vi "Stop.vi"(8 "error in (no error)":errorcluster, 10 "Message in":refnum<class "StopMessage.lvclass">, 11 "Autofocus in":refnum<class "Autofocus.lvclass">) -> (0 "error out":errorcluster, 3 "Autofocus out":refnum<class "Autofocus.lvclass">)   [LabVIEW 2012, in "Autofocus.lvclass"]
doc: "This member function is called when the statemachine in the run.vi receives an 'stop' command. It relays the message to all observers of the component.\n\nOverride this member function in your derived class if you need additional stop functionality (but don't forget to call the parent method)."
uses:
  Autofocus.lvclass
  <vilib>/Distrio/Murmex/StopMessage/StopMessage.lvclass
  <vilib>/Distrio/Murmex/Murmex/Murmex.lvclass
  Autofocus.lvclass/Autofocus.ctl
panel:
  out "optimisation duration":dbl
  # "This method is called when the STOP\ntrigger is sent. \n\nOverride this method when your component needs to\nrespond to this trigger. \n\nCall parent for proper implementation"
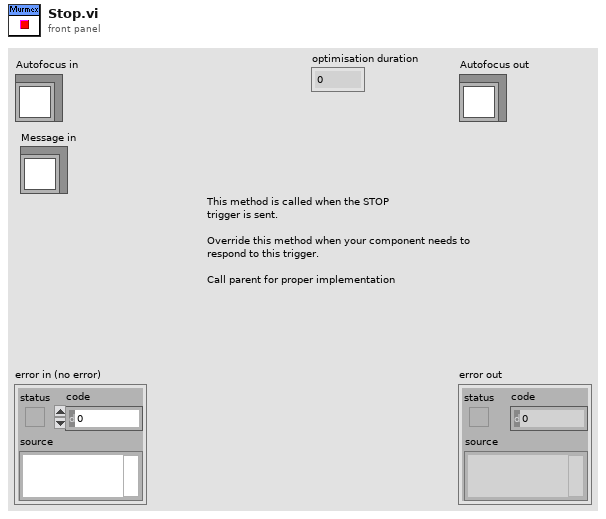
[diagram p1: front panel]
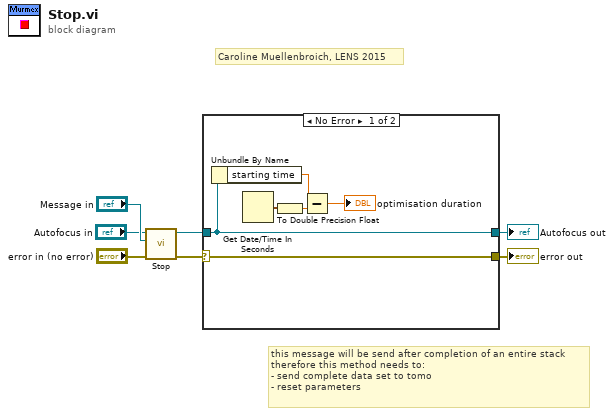
[diagram p0: block diagram]
diagram:
  # "Caroline Muellenbroich, LENS 2015"
  # "this message will be send after completion of an entire stack\ntherefore this method needs to:\n- send complete data set to tomo\n- reset parameters"
  n1 = call-parent "Stop.vi"("error in (no error)"="error in (no error)", "Message in"="Message in", "Murmex in"="Autofocus in") -> ("error out"=w4:errorcluster, "Murmex out"=w3:refnum<class "Autofocus.lvclass">)  [unwired: 7 in]
  n2 = case shown="No Error" w4 {
    selector: w4 -> [w11 w15]
    tunnel: w3 -> [w12 w14]
    tunnel: [w11 w15] -> w2
    tunnel: [w12 w14] -> w1
    frame No Error {
      n3 = Unbundle By Name(w12) -> ("starting time"=w10:dbl)
      n4 = Get Date/Time In Seconds() -> (seconds since 1Jan1904=w13:timestamp)
      n5 = To Double Precision Float(number=w13) -> (double precision float=w9:dbl)
      n6 = Subtract(x=w10, y=w9) -> (x-y=→"optimisation duration":dbl)
    }
    frame Error {
    }
  }
  "error out" <- w2
  "Autofocus out" <- w1
